vi "html.vi"   [LabVIEW 2015]
uses:
  <vilib>/nao/NAO SDK.lvlib
types:
  T1 = typedef "NAO SDK.lvlib/TabletServiceRef.ctl" = refnum<k1>
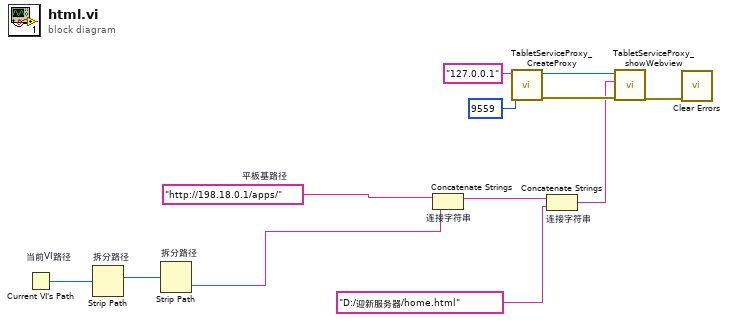
[diagram p0: block diagram]
diagram:
  w3 = "http://198.18.0.1/apps/"  # 平板基路径
  n1 = Current VI's Path "当前VI路径"() -> (path=w4:path)
  n2 = Strip Path "拆分路径"(path=w4) -> (stripped path=w5:path)  [unwired: 1 out]
  n3 = Strip Path "拆分路径"(path=w5) -> (name=w1:string)  [unwired: 1 out]
  n4 = Concatenate Strings "连接字符串"(w3, w1) -> (w6:string)
  n5 = call <vilib>:"TabletServiceProxy_CreateProxy.vi"("pPort"=9559, "pIP"="127.0.0.1") -> ("ErrorOut"=w9:errorcluster, "TabletServiceRef"=w10:T1)  [unwired: 8 in]
  n6 = Concatenate Strings "连接字符串"(w6, "D:/迎新服务器/home.html" ("字符串")) -> (w7:string)
  n7 = call <vilib>:"TabletServiceProxy_showWebview.vi"("ErrorIn"=w9, "Webview"=w7, "TabletService"=w10) -> ("ErrorOut"=w8:errorcluster)  [unwired: 7 in, 1 out]
  n8 = call <vilib>:"Clear Errors.vi"("error in (no error)"=w8) -> ()  [unwired: 5 in, 2 out]
